vi "Position First Numeric.vi"(8 "error in (no error)":errorcluster, 10 "Button Ref":refnum<vi>, 11 "Numeric Ref":refnum<vi>) -> (0 "Error Out":errorcluster)   [LabVIEW 2014]
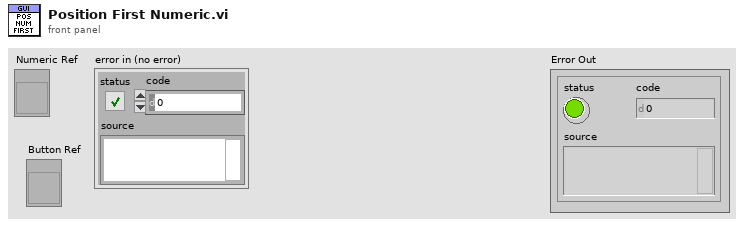
[diagram p1: front panel]
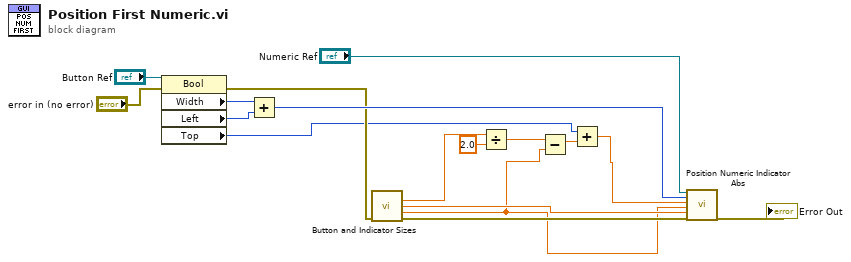
[diagram p0: block diagram]
diagram:
  n1 = property class="Bool"(reference="Button Ref", error in="error in (no error)") -> (error out=w9:errorcluster, "Width"=w12:u32, "Left"=w11:i32, "Top"=w4:i32)  [unwired: 1 out]
  n2 = Add(x=w12, y=w11) -> (x+y=w10:u32)
  n3 = call "Button and Indicator Sizes.vi"("error in (no error)"=w9) -> ("Button Height"=w7:dbl, "Numerice Indicator Width"=w15:dbl, "Numeric Indicator Height"=w1:dbl, "error out"=w16:errorcluster)  [unwired: 10 in, 1 out]
  n4 = Divide(x=w7, y=2.0) -> (x/y=w6:dbl)
  n5 = Subtract(x=w6, y=w1) -> (x-y=w3:dbl)
  n6 = Add(x=w4, y=w3) -> (x+y=w2:dbl)
  n7 = call "Position Numeric Indicator Abs.vi"("Numeric Ref"="Numeric Ref", "Left Offset (px)"=w10, "Top Offste (px)"=w2, "Height (px)"=w1, "Width (px)"=w15, "Error In"=w16) -> ("Error Out"=→"Error Out":errorcluster)  [unwired: 13 in]
